vi "DCA Compute T-Zout.vi"(1 "Measurement Values":T1) -> (0 "T-Zout":dbl)   [LabVIEW 2011]
uses:
  TypeDefs/DCA Measurement Values.ctl
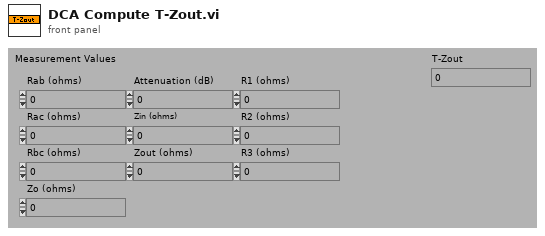
[diagram p1: front panel]
types:
  T1 = typedef "DCA Measurement Values.ctl" = cluster{"Rab (ohms)":dbl, "Rac (ohms)":dbl, "Rbc (ohms)":dbl, "Zo (ohms)":dbl, "Attenuation (dB)":dbl, "Zin (ohms)":dbl, "Zout (ohms)":dbl, "R1 (ohms)":dbl, "R2 (ohms)":dbl, "R3 (ohms)":dbl}
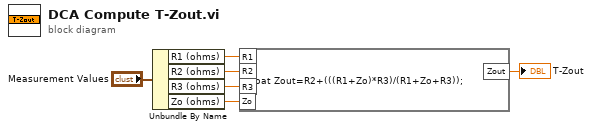
[diagram p0: block diagram]
diagram:
  n1 = Unbundle By Name("Measurement Values") -> ("R1 (ohms)"=w5:dbl, "R2 (ohms)"=w4:dbl, "R3 (ohms)"=w3:dbl, "Zo (ohms)"=w1:dbl)
  n2 = formula code="float Zout=R2+(((R1+Zo)*R3)/(R1+Zo+R3));"("R1"=w5, "R2"=w4, "R3"=w3, "Zo"=w1) -> ("Zout"=→"T-Zout":dbl)
